vi "Grove Read ADC.vi"() -> ()   [LabVIEW 2020, in "CTI-Scratchpad.lvlib"]
uses:
  CTI-Scratchpad.lvlib
  CTI/Error Reporting.ctl
  CTI/Identity.ctl
  CTI/ADC Number.ctl
  CTI/Session/Session.lvclass
  CTI/CTI.lvlib
  CTI/VisaComms/VisaComms.lvclass
panel:
  out "Identity":T1
  in  "GroveConnector":enum16{"A0", "A1", "A2"}(ring)
  in  "Error Checking (Full)":T2
  in  "Speed":i32(slide)=12 scale=1000.0..1.0
  in  "stop":bool
  out "ADC":u16(graph)
  in  "Port":refnum<visa-resource-name>="TCPIP::10.190.177.58::5555::SOCKET"
  # "https://wiki.seeedstudio.com/Grove-Rotary_Angle_Sensor/#version"
  # "https://wiki.seeedstudio.com/Grove-2.5A-DC-Current-Sensor-ACS70331/"
  # "https://wiki.seeedstudio.com/Grove-5A_DC_AC_Current_Sensor-ACS70331/"
  # "https://wiki.seeedstudio.com/Grove-10A_DC_Current_Sensor-ACS725/"
  # "https://wiki.seeedstudio.com/Grove-Air_Quality_Sensor_v1.3/"
  # "https://wiki.seeedstudio.com/Grove-Round_Force_Sensor_FSR402/"
  # "https://wiki.seeedstudio.com/Grove-Capacitive_Moisture_Sensor-Corrosion-Resistant/"
  # "https://wiki.seeedstudio.com/Grove-Slide_Potentiometer/"
  # "https://wiki.seeedstudio.com/Grove-EC-Sensor-kit/"
  # "https://wiki.seeedstudio.com/Grove-TDS-Sensor/"
  # "http://wiki.seeedstudio.com/Grove-Turbidity-Sensor-Meter-for-Arduino-V1.0/"
  # "https://wiki.seeedstudio.com/Grove-Temperature_Sensor/"
  # "https://wiki.seeedstudio.com/Grove-Loudness_Sensor/"
  # "https://wiki.seeedstudio.com/Grove-Voltage_Divider/"
  # "https://wiki.seeedstudio.com/Grove-Luminance_Sensor/"
  # "https://wiki.seeedstudio.com/Grove-Gas_Sensor-MQ2/"
  # "https://wiki.seeedstudio.com/Grove-Moisture_Sensor/"
  # "https://wiki.seeedstudio.com/Grove-Gas_Sensor-MQ3/"
  # "https://wiki.seeedstudio.com/Grove-ORP-Sensor-kit/"
  # "https://wiki.seeedstudio.com/Grove-Gas_Sensor-MQ5/"
  # "https://wiki.seeedstudio.com/Grove-PH-Sensor-kit/"
  # "https://wiki.seeedstudio.com/Grove-Gas_Sensor-MQ9/"
  # "https://wiki.seeedstudio.com/Grove-Gas_Sensor-O2/"
  # "https://wiki.seeedstudio.com/Grove-Gas_Sensor-O2-MIX8410/"
  # "https://wiki.seeedstudio.com/Grove-High_Temperature_Sensor/"
  # "https://wiki.seeedstudio.com/Grove-Infrared_Temperature_Sensor/"
  # "https://wiki.seeedstudio.com/Grove-Light_Sensor/#upgradable-to-industrial-sensors"
  # "https://www.seeedstudio.com/Grove-Sound-Sensor-Based-on-LM358-amplifier-Arduino-Compatible.html"
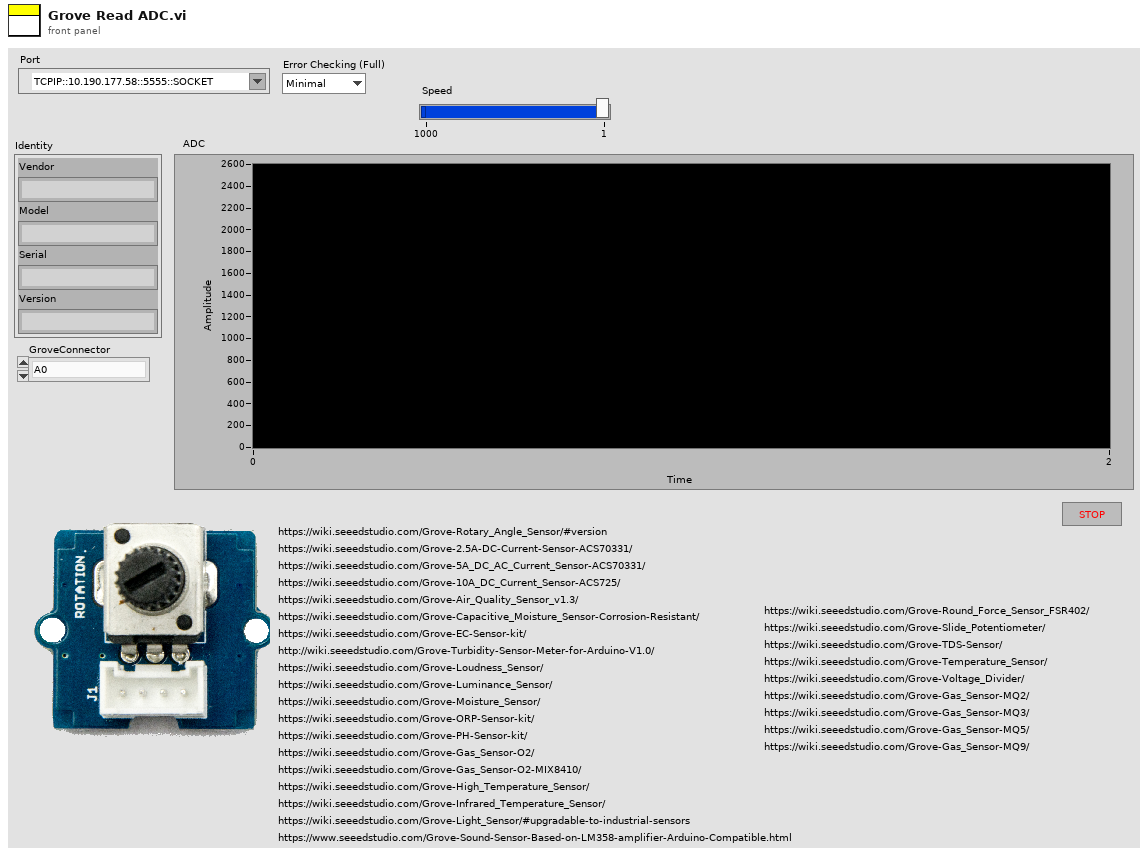
[diagram p1: front panel]
types:
  T1 = typedef "CTI.lvlib/Identity.ctl" = cluster{"Vendor":string, "Model":string, "Serial":string, "Version":string}
  T2 = typedef "CTI.lvlib/Error Reporting.ctl" = enum16{"Minimal", "Moderate", "Full"}
  T3 = typedef "CTI.lvlib/ADC Number.ctl" = i8
  T4 = typedef "CTI.lvlib/Raw ADC.ctl" = u16
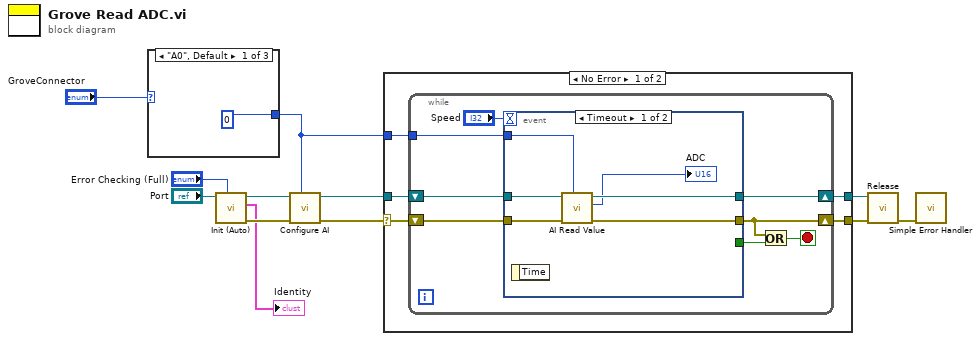
[diagram p0: block diagram]
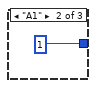
[diagram p2: hidden frame]
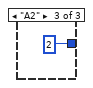
[diagram p3: hidden frame]
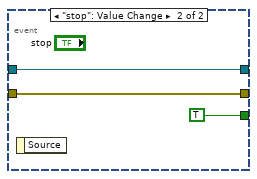
[diagram p4: hidden frame]
diagram:
  n1 = case shown="\"A0\", Default" "GroveConnector" {
    tunnel: [T3 0 T3 1 T3 2] -> w1
    frame "A0", Default {
    }
    frame "A1" {
    }
    frame "A2" {
    }
  }
  n2 = call "Init (Auto).vi"("Error Checking (Full)"="Error Checking (Full)", "VISA resource name"="Port") -> ("error out"=w10:errorcluster, "Identity"=→"Identity":T1, "Session"=w11:refnum<class "Session.lvclass">)  [unwired: 7 in]
  n3 = call "Configure AI.vi"("ADC #"=w1, "error in (no error)"=w10, "Session in"=w11) -> ("error out"=w9:errorcluster, "Session out"=w8:refnum<class "Session.lvclass">)  [unwired: 7 in]
  n4 = case shown="No Error" w9 {
    selector: w9 -> [w18 w39]
    tunnel: w8 -> [w19 w38]
    tunnel: w1 -> [w20 _]
    tunnel: [w16 w39] -> w6
    tunnel: [w17 w38] -> w7
    frame No Error {
      n5 = while {
        tunnel: w20 -> [w27]
        shift-right: [w24] -> w17
        shift-left: w19 -> [w26]
        shift-right: [w23] -> w16
        shift-left: w18 -> [w25]
        stop <- w21 stop-if-true
        n6 = event shown="[0] Timeout" {
          selector: _ -> [_ _]
          dyn-events: _ -> [_ _]
          timeout: "Speed" -> [_ _]
          tunnel: w27 -> [w32 _]
          tunnel: w26 -> [w34 w35]
          tunnel: w25 -> [w33 w36]
          tunnel: [w31 w35] -> w24
          tunnel: [w30 w36] -> w23
          tunnel: [_ TRUE] -> w22
          event Timeout {
            n7 = event-data() -> ()  [unwired: 1 in, 1 out]
            n8 = call "AI Read Value.vi"("ADC #"=w32, "error in (no error)"=w33, "Session in"=w34) -> ("error out"=w30:errorcluster, "Value"=→"ADC":T4, "Session out"=w31:refnum<class "Session.lvclass">)  [unwired: 6 in]
          }
          event "stop": Value Change {
            n9 = event-data() -> ()  [unwired: 1 in, 1 out]
          }
        }
        n10 = Or(x=w23, y=w22) -> (x .or. y?=w21:bool)
      }
    }
    frame Error {
    }
  }
  n11 = call-dynamic "Release.vi"("error in (no error)"=w6, "Session in"=w7) -> ("error out"=w5:errorcluster)  [unwired: 9 in]
  n12 = call <vilib>:"Simple Error Handler.vi"("error in (no error)"=w5) -> ()  [unwired: 4 in, 5 out]
